vi "Log String.vi"(5 "Level":T1, 6 "String":string, 8 "error in (no error)":errorcluster, 11 "Application Log in":refnum<class "Application Log.lvclass">) -> (0 "error out":errorcluster, 3 "Application Log out":refnum<class "Application Log.lvclass">)   [LabVIEW 2016, in "Stream Log.lvlib" / "Application Log.lvclass"]
doc: "--\nCopyright © 2017 Composed SystemsI All rights reserved.\n\nAuthor: Jon McBee <jon.mcbee@composed.io>\n\nThis library is provided \"AS IS\" ,WITHOUT WARRANTIES OR\nCONDITIONS OF ANY KIND, either express or implied.\n\nComposed Systems -- composed.io\n\nStream 0.0.1.1\nJon McBee - Composed Systems\nCopyright (c) 2017, Composed Systems"
uses:
  <userlib>/Composed Systems/Stream/Log/Application Log/Application Log.lvclass
  <userlib>/Composed Systems/Stream/Log/Application Log/Log Level.ctl
  <userlib>/Composed Systems/Stream/Log/Application Log/Application Log.lvclass/Application Log.ctl
  <userlib>/Composed Systems/Stream/Log/Sink Look Up Table/Sink Look Up Table.lvclass
  C:/Program Files (x86)/National Instruments/LabVIEW 2016/user.lib/Composed Systems/Stream/Look Up Table/Look Up Table/Look Up Table.lvclass
  <userlib>/Composed Systems/Stream/Log/Log Sink/Log Sink.lvclass
  <userlib>/Composed Systems/Stream/Look Up Table/Look Up Table/Look Up Table.lvclass
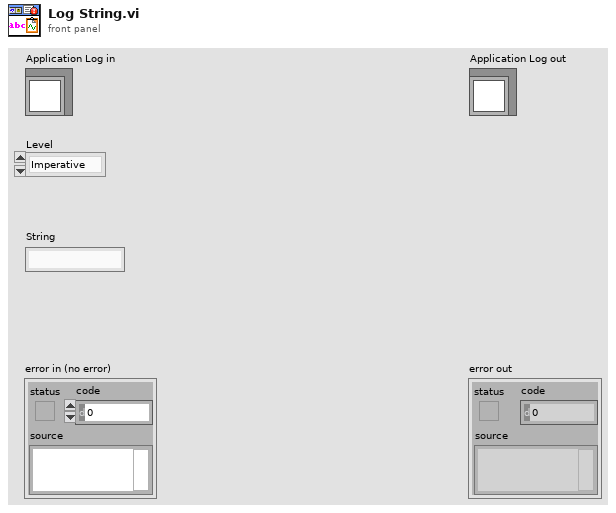
[diagram p1: front panel]
types:
  T1 = typedef "Stream Log.lvlib/Application Log.lvclass/Log Level.ctl" = enum16{"Imperative", "Major", "Minor", "Debug", "Off"}
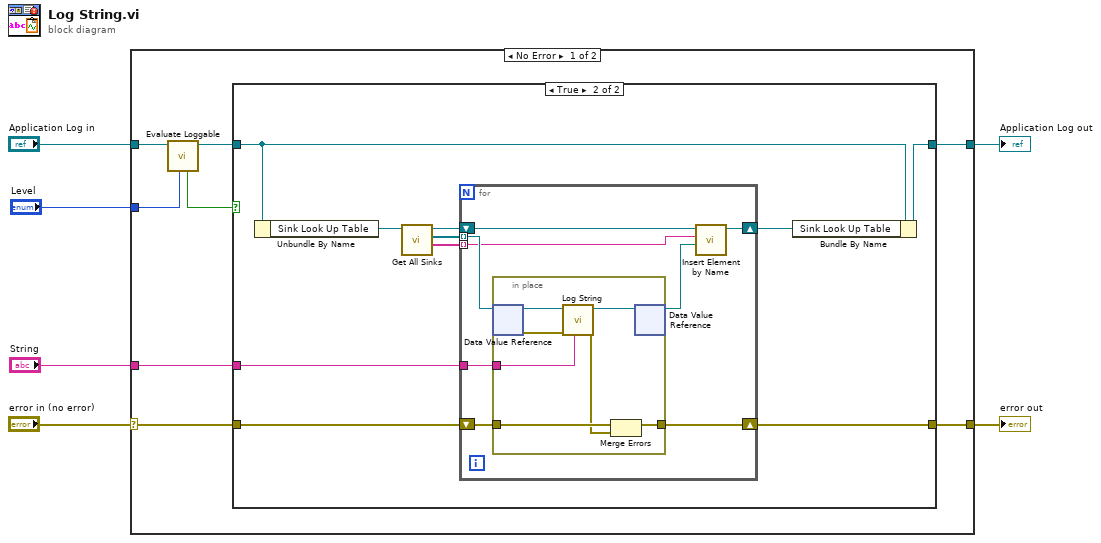
[diagram p0: block diagram]
diagram:
  n1 = case shown="No Error" "error in (no error)" {
    selector: "error in (no error)" -> [w9 w43]
    tunnel: [w8 w43] -> w5
    tunnel: [w10 w42] -> w3
    tunnel: "Application Log in" -> [w14 w42]
    tunnel: "Level" -> [w13 _]
    tunnel: "String" -> [w7 _]
    frame No Error {
      n2 = call <userlib>:"Evaluate Loggable.vi"("Level"=w13, "Application Log in"=w14) -> ("Application Log out"=w11:refnum<class "Application Log.lvclass">, "Log?"=w12:bool)  [unwired: 8 in]
      n3 = case shown="True" w12 {
        tunnel: [w16 w22] -> w10
        tunnel: w11 -> [w16 w23]
        tunnel: [w15 w25] -> w8
        tunnel: w9 -> [w15 w26]
        tunnel: w7 -> [_ w24]
        frame False {
        }
        frame True {
          n4 = Unbundle By Name(w23) -> ("Sink Look Up Table"=w21:refnum<class "Sink Look Up Table.lvclass">)
          n5 = call <userlib>:"Get All Sinks.vi"("Sink Look Up Table in"=w21) -> ("Names"=w18:string[], "Sinks"=w20:refnum<data-value>[], "Sink Look Up Table out"=w19:refnum<class "Sink Look Up Table.lvclass">)  [unwired: 7 in, 1 out]
          n6 = for {
            shift-right: [w31] -> w25
            shift-left: w26 -> [w32]
            tunnel: w20 -> [w34] mode=indexing
            tunnel: w24 -> [w33]
            shift-right: [w29] -> w17
            shift-left: w19 -> [w30]
            tunnel: w18 -> [w28] mode=indexing
            n7 = in-place {
              in-place-border: w33 -> [w38]
              in-place-border: w32 -> [w37]
              in-place-border: [w35] -> w31
              n8 = in-place-dvr #1(w34) -> (w41:refnum<class "Log Sink.lvclass">, w39:errorcluster)
              n9 = call-dynamic "Log String.vi"("String"=w38, "error in (no error)"=w39, "Log Sink in"=w41) -> ("error out"=w36:errorcluster, "Log Sink out"=w40:refnum<class "Log Sink.lvclass">)  [unwired: 7 in]
              n10 = Merge Errors(w37, w36) -> (w35:errorcluster)
              n11 = in-place-dvr #1(w40) -> (w27:refnum<data-value>)  [unwired: 1 out]
            }
            n12 = call <userlib>:"Insert Element by Name.vi"("Variant"=w27, "Name"=w28, "Look Up Table in"=w30) -> ("Look Up Table out"=w29:refnum<class "Sink Look Up Table.lvclass">)  [unwired: 6 in, 2 out]
          }
          n13 = Bundle By Name(cluster=w23, "Sink Look Up Table"=w17) -> (w22:refnum<class "Application Log.lvclass">)
        }
      }
    }
    frame Error {
    }
  }
  "error out" <- w5
  "Application Log out" <- w3
